vi "Main.vi"() -> ()   [LabVIEW 2022 SP3]
panel:
  in  "Waiting Time":dbl
  in  "Number 4":dbl
  in  "Number 3":dbl
  out "Result 2":dbl
  out "Result 1":dbl
  in  "Number 2":dbl
  in  "Number 1":dbl
  # "="
  # "+"
  # "-"
  # "="
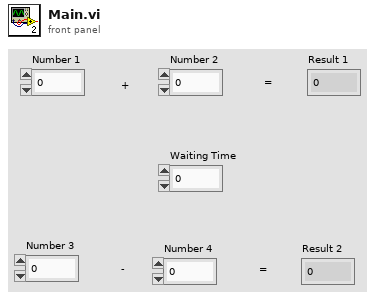
[diagram p1: front panel]
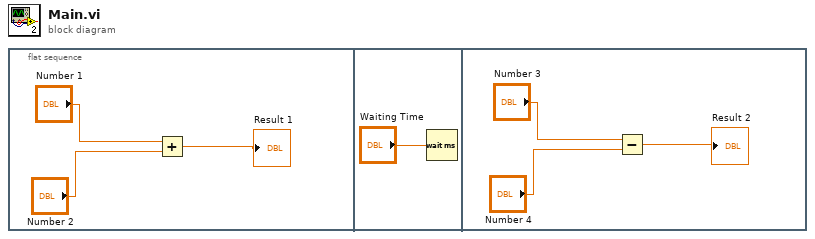
[diagram p0: block diagram]
diagram:
  n1 = flat-sequence {
    frame #0 {
      n2 = Add(x="Number 1", y="Number 2") -> (x+y=→"Result 1":dbl)
    }
    frame #1 {
      n3 = Wait (ms)(milliseconds to wait="Waiting Time") -> ()  [unwired: 1 out]
    }
    frame #2 {
      n4 = Subtract(x="Number 3", y="Number 4") -> (x-y=→"Result 2":dbl)
    }
  }
